vi "Robot Global Data.vi"() -> ()   [LabVIEW 2019]
doc: "This global VI can contain as many global variables as you need. Place a control on the panel, give it a good name. To read or write to it from a VI, drag the icon to the diagram of that VI. You can also drag from the project. Click on the node to change which global you access. You shouldn't have multiple locations writing to a global or it will cause a race-condition."
uses:
  <vilib>/Rock Robotics/WPI/Camera/WPI_CameraImageSize.ctl
  <vilib>/Rock Robotics/WPI/DriverStation/WPI_DriverStationRobotMode2.ctl
panel:
  out "Auto Move Num":dbl
  out "Auto R":dbl
  out "Auto L":dbl
  out "Bottom RPM":dbl
  out "Top RPM":dbl
  out "Distance":dbl
  out "RS - Y":dbl
  out "RS - X":dbl
  out "BUT 12":bool
  out "BUT 11":bool
  out "BUT 10":bool
  out "BUT 9":bool
  out "BUT 7":bool
  out "BUT 6":bool
  out "BUT 5":bool
  out "BUT 4":bool
  out "BUT 3":bool
  out "BUT 2":bool
  out "BUT 1":bool
  out "BUT 8":bool
  out "TS":dbl
  out "TA":dbl
  out "TY":dbl
  out "TX":dbl
  out "Joystick Y":dbl
  out "Joystick X":dbl
  in  "Robot Mode":T1
  in  "image size":T2=enum."320x240"
  in  "Enable Vision":bool
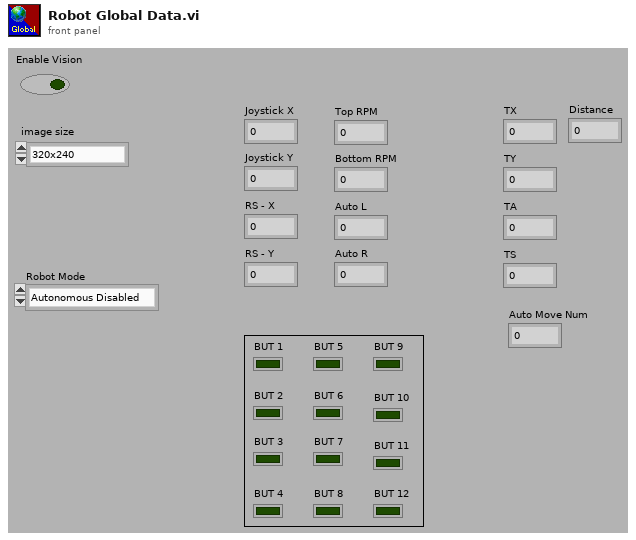
[diagram p1: front panel]
types:
  T1 = typedef "WPI_DriverStationRobotMode2.ctl" = enum16{"Autonomous Disabled", "Autonomous Enabled", "Teleop Disabled", "Teleop Enabled", "Disconnected", "Finish", "Test Disabled", "Test Enabled", "Emergency Stopped"}
  T2 = typedef "WPI_CameraImageSize.ctl" = enum16{"640x480", "320x240", "160x120", "Custom"}
diagram:
